vi "Zadanie 5.vi"() -> ()   [LabVIEW 2020]
panel:
  out "p>q":bool
  out "p=q":bool
  in  "q":u8
  in  "p":u8
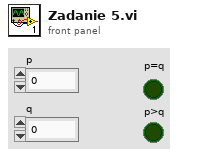
[diagram p1: front panel]
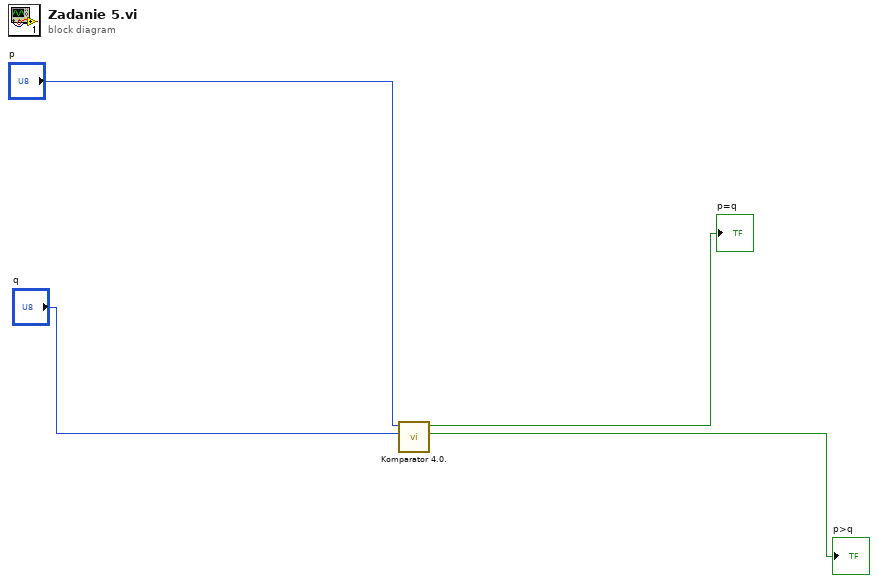
[diagram p0: block diagram]
diagram:
  n1 = call "Komparator 4.0..vi"("Q"="q", "P"="p") -> ("P>Q"=→"p>q":bool, "P=Q"=→"p=q":bool)  [unwired: 8 in]
